vi "WS1021 Multi DUT Verify Beam RB.vi"(6 "FPGA":T1, 8 "Error In":errorcluster, 11 "Register RB":string[](array[string])=["0762", "0763"]) -> (0 "Error Out":errorcluster, 2 "Board B":string[][](array[string]), 3 "Board A":string[][](array[string]))   [LabVIEW 2017]
uses:
  WS_VCAP Driver 039/Source/WSVCAP Shell/Type Defs/WSVCAP SHL FPGA Enum.ctl
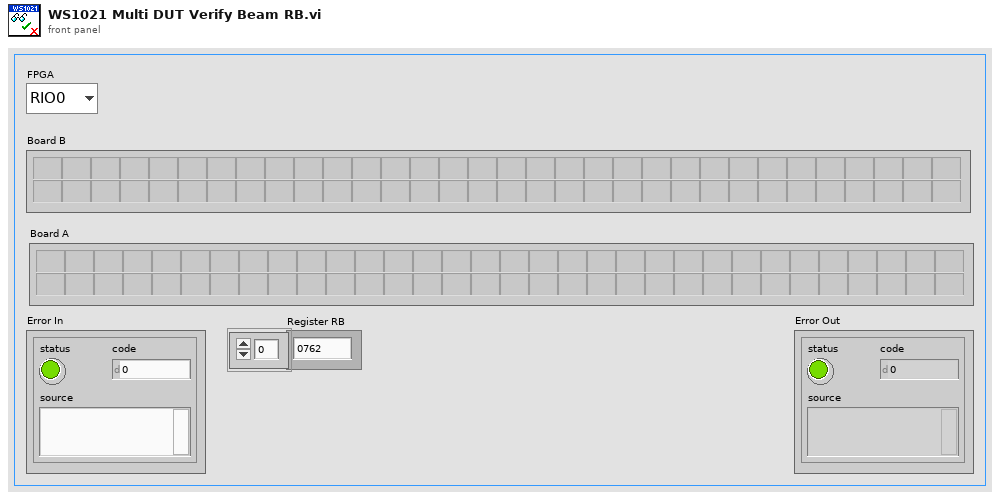
[diagram p1: front panel]
types:
  T1 = typedef "WSVCAP SHL FPGA Enum.ctl" = enum16{"RIO0", "RIO1"}
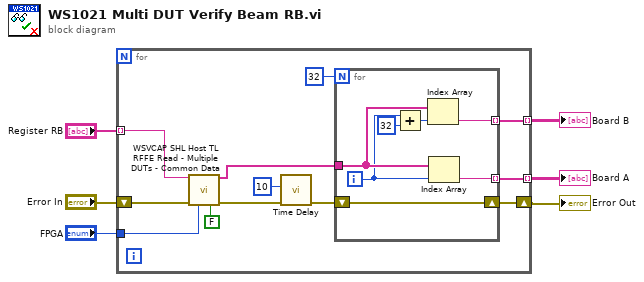
[diagram p0: block diagram]
diagram:
  n1 = for {
    tunnel: "Register RB" -> [w17] mode=indexing
    tunnel: "FPGA" -> [w16]
    shift-right: [w10] -> w1
    shift-left: "Error In" -> [w18]
    tunnel: [w8] -> w4 mode=indexing
    tunnel: [w7] -> w3 mode=indexing
    n2 = call "WSVCAP SHL Host TL RFFE Read - Multiple DUTs - Common Data.vi"("Data Out"=w17, "error in"=w18, "FPGA"=w16, "Log (T)"=FALSE) -> ("RFFE Data In"=w9:string[], "error out"=w14:errorcluster)  [unwired: 10 in]
    n3 = call "Time Delay.vi"("Error In"=w14, "Delay(ms)"=u32 10) -> ("Error Out"=w11:errorcluster)  [unwired: 9 in]
    n4 = for {
      N: 32 -> [_]
      shift-right: [w25] -> w10
      shift-left: w11 -> [w25]
      tunnel: w9 -> [w24]
      tunnel: [w20] -> w8 mode=indexing
      tunnel: [w19] -> w7 mode=indexing
      i -> [w22]
      n5 = Add(x=w22, y=32) -> (x+y=w23:i32)
      n6 = Index Array(array=w24, index=w23) -> (element=w20:string)
      n7 = Index Array(array=w24, index=w22) -> (element=w19:string)
    }
  }
  "Board B" <- w4
  "Board A" <- w3
  "Error Out" <- w1
